vi "format set bottom color.vi"(8 "error in (no error)":errorcluster, 10 "color":u32, 11 "format":u32) -> (0 "error out":errorcluster)   [LabVIEW 2015, in "xlsxwriter.lvlib"]
doc: "void format_set_bottom_color(lxw_format format, lxw_color_t color);"
uses:
  xlsxwriter.lvlib
  xlsxwriter.dll
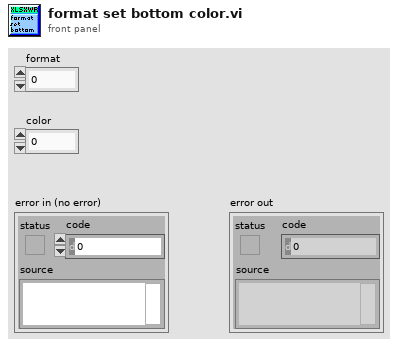
[diagram p1: front panel]
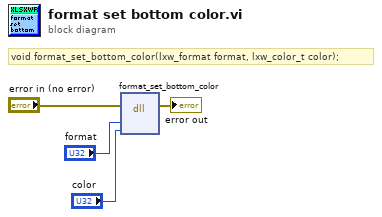
[diagram p0: block diagram]
diagram:
  # "void format_set_bottom_color(lxw_format format, lxw_color_t color);"
  n1 = dll-call lib="C:/Users/WDAGUtilityAccount/Desktop/lv_vis_added_cell/xlsxwriter.*" fn="format_set_bottom_color"(error in="error in (no error)", "format"="format", "color"="color") -> (error out=→"error out":errorcluster)  [unwired: 5 in, 1 out]
